vi "test_SessionsReserved_CallUnreserveSessions_AllowsSessionsToBeReservedAgain.vi"(8 "error in":errorcluster) -> (0 "error out":errorcluster, 2 "result":string, 3 "pass":bool)   [LabVIEW 2020, in "MeasurementServerTests.lvlib"]
uses:
  MeasurementServerTests.lvlib
  Runtime/MeasurementLink Session Management/Session Reservation/Session Reservation.lvclass
  Runtime/MeasurementLink Session Management Client/RPC Messages/ni_measurementlink_PinMapContext.ctl
  Runtime/MeasurementLink Session Management Client/MeasurementLink Session Management Client.lvlib
  Helpers/Pin Map XML Strings Global.vi
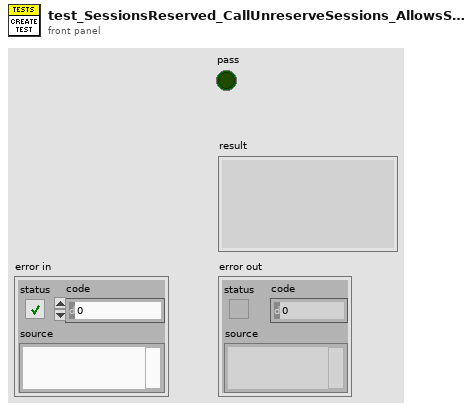
[diagram p1: front panel]
types:
  T1 = typedef "MeasurementLink Session Management Client.lvlib/ni_measurementlink_PinMapContext.ctl" = cluster{"pin_map_id":string, "sites":i32[]}
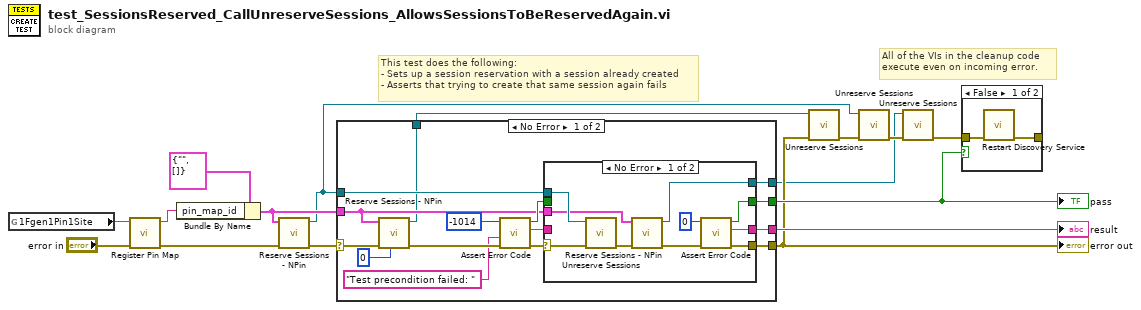
[diagram p0: block diagram]
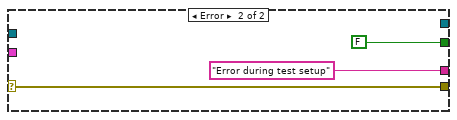
[diagram p3: hidden frame]
diagram:
  # "All of the VIs in the cleanup code\nexecute even on incoming error."
  # "This test does the following:\n- Sets up a session reservation with a session already created\n- Asserts that trying to create that same session again fails"
  n1 = global read "Pin Map XML Strings Global.vi" "1Fgen1Pin1Site"() -> (w10:string)
  n2 = call "Register Pin Map.vi"("error in"="error in", "pin map xml"=w10) -> ("error out"=w13:errorcluster, "pin map id"=w11:string)  [unwired: 8 in]
  n3 = Bundle By Name(cluster=T1 {"pin_map_id"="", "sites"=[]} ("pin map context"), "pin_map_id"=w11) -> (w7:T1)
  n4 = call "Reserve Sessions - NPin.vi"("error in"=w13, "pin map context"=w7) -> ("error out"=w8:errorcluster, "session reservation out"=w4:refnum<class "Session Reservation.lvclass">)  [unwired: 8 in]
  n5 = case shown="No Error" w8 {
    selector: w8 -> [w28 w45]
    tunnel: [w26 w45] -> w14
    tunnel: [w23 FALSE] -> w15
    tunnel: [w25 "Error during test setup" ("f")] -> w16
    tunnel: w7 -> [w19 _]
    tunnel: w4 -> [w20 _]
    tunnel: [w18 _] -> w3
    tunnel: [w17 _] -> w1
    frame No Error {
      n6 = call "Reserve Sessions - NPin.vi"("timeout (ms)"=0, "error in"=w28, "pin map context"=w19) -> ("error out"=w31:errorcluster, "session reservation out"=w17:refnum<class "Session Reservation.lvclass">)  [unwired: 7 in]
      n7 = call "Assert Error Code.vi"("error in"=w31, "additional info to prepend"="Test precondition failed: ", "expected error code"=-1014) -> ("error out"=w27:errorcluster, "details"=w24:string, "error code match?"=w22:bool)  [unwired: 6 in]
      n8 = case shown="No Error" w27 {
        selector: w27 -> [w41 w44]
        tunnel: [w35 w44] -> w26
        tunnel: [w34 w43] -> w25
        tunnel: w24 -> [_ w43]
        tunnel: [w33 w42] -> w23
        tunnel: w22 -> [_ w42]
        tunnel: w20 -> [w40 _]
        tunnel: w19 -> [w38 _]
        tunnel: [w32 _] -> w18
        frame No Error {
          n9 = call "Unreserve Sessions.vi"("error in"=w41, "session reservation in"=w40) -> ("error out"=w39:errorcluster)  [unwired: 9 in]
          n10 = call "Reserve Sessions - NPin.vi"("error in"=w39, "pin map context"=w38) -> ("error out"=w36:errorcluster, "session reservation out"=w32:refnum<class "Session Reservation.lvclass">)  [unwired: 8 in]
          n11 = call "Assert Error Code.vi"("error in"=w36, "expected error code"=0) -> ("error out"=w35:errorcluster, "details"=w34:string, "error code match?"=w33:bool)  [unwired: 7 in]
        }
        frame Error {
        }
      }
    }
    frame Error {
    }
  }
  "error out" <- w14
  "pass" <- w15
  "result" <- w16
  n12 = call "Unreserve Sessions.vi"("error in"=w14, "session reservation in"=w1) -> ("error out"=w2:errorcluster)  [unwired: 9 in]
  n13 = call "Unreserve Sessions.vi"("error in"=w2, "session reservation in"=w4) -> ("error out"=w6:errorcluster)  [unwired: 9 in]
  n14 = call "Unreserve Sessions.vi"("error in"=w6, "session reservation in"=w3) -> ("error out"=w5:errorcluster)  [unwired: 9 in]
  n15 = case shown="False" w15 {
    tunnel: w5 -> [w49 _]
    tunnel: [w48 _] -> _
    frame False {
      n16 = call "Restart Discovery Service.vi"("error in"=w49) -> ("error out"=w48:errorcluster)  [unwired: 10 in]
    }
    frame True {
    }
  }
